vi "Adjust_Library_URL.vi"(8 "error in (no error)":errorcluster, 9 "libray ref":refnum<vi>, 10 "source path":path, 11 "Build in":refnum<class "AB_EXE.lvclass">) -> (0 "error out":errorcluster, 3 "Build out":refnum<class "AB_EXE.lvclass">)   [LabVIEW 2020, in "AB_EXE.lvclass"]
uses:
  <vilib>/AppBuilder/AB_Classes/EXE/AB_EXE.lvclass
  e:/builds/penguin/labview/branches/2020/dev/dist/vi.lib/AppBuilder/AB_Classes/Build/AB_Build.lvclass
  <vilib>/AppBuilder/AB_Classes/EXE/AB_EXE.lvclass/AB_EXE.ctl
  <vilib>/AppBuilder/AB_Classes/Build/AB_Build.lvclass
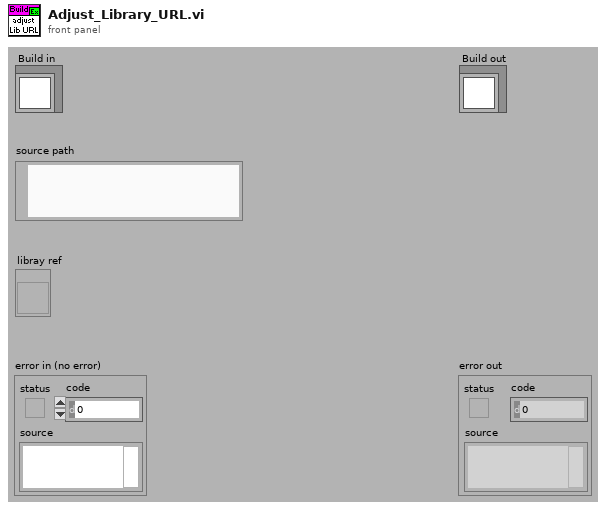
[diagram p1: front panel]
types:
  T1 = typedef "AB_EXE_SharedVar_LibInfo.ctl" = cluster{"LibraryPath":path, "LibraryItemID":string, "target":string, "deploy":bool}
  T2 = typedef "AB_Build.ctl" = cluster{"buildSpecName":string, "buildSpecDescription":string, "destinations":refnum<class "AB_Destination.lvclass">[], "exclusionOption":T3, "defaultLanguage":string, "supportedLanguages":string[], "excludedDirectories":path[], "buildContext":refnum<vi>, "buildObject":T4, "preview":bool, "programatic":bool, "progressBarEvents":T5, "userLog_Path":path, "preActionID":string, "preAction_Path":path, "postActionID":string, "postAction_Path":path, "eng_checkForBrokenVIs?":bool, "eng_verboseLinkerErrors?":bool, "localDest_Path":path, "targetDest_Path":path, "removeVIObject":u16, "cache":refnum<class "PreviewCache.lvclass">, "use cache":bool, "previewCache_ID":string, "buildCache_ID":string, "eng_TempLocalDest_Path":path, "eng_collectDependencies?":bool, "versionInfo":cluster{"buildVersion":cluster{"major":u16, "minor":u16, "patch":u16, "build":u16}, "autoIncrement":bool}, "eng_enableVIChecksums":bool}
  T3 = typedef "AB_Exclusion_Option.ctl" = cluster{"typedefs":bool, "polymorphicVIs":bool, "unusedLibraryItems":bool, "modifyLibraryFile":bool, "edit-timeDependencies":bool, "inlineVIs":bool, "dependent PPLs":bool, "dependent DLLs":bool}
  T4 = typedef "ItemRef.ctl" = u64
  T5 = typedef "provcom_ProgressBar_Events.ctl" = cluster{"newJob":refnum<user-event>, "newItem":refnum<user-event>, "errorMsg":T6, "cancel":refnum<user-event>}
  T6 = typedef "mxLvBuildError.ctl" = refnum<user-event>
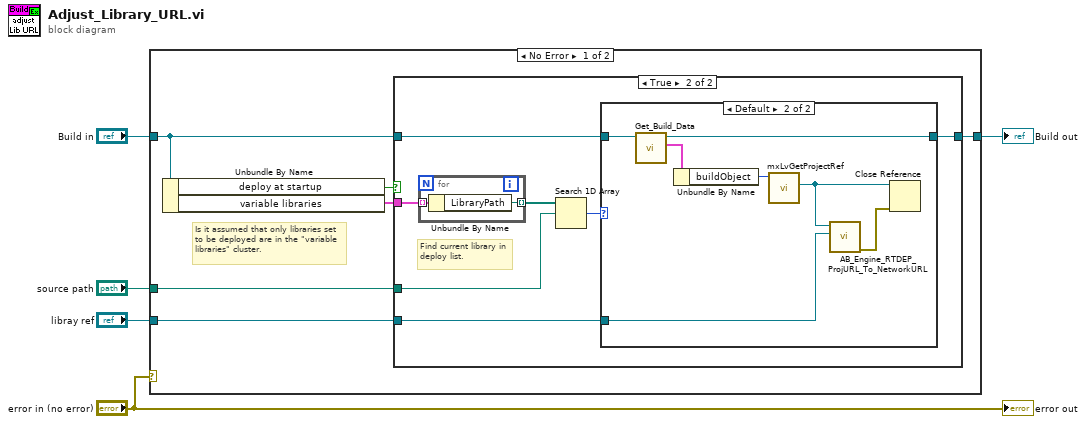
[diagram p0: block diagram]
diagram:
  n1 = case shown="No Error" "error in (no error)" {
    tunnel: "Build in" -> [w11 w30]
    tunnel: [w9 w30] -> w4
    tunnel: "source path" -> [w7 _]
    tunnel: "libray ref" -> [w6 _]
    frame No Error {
      # "Is it assumed that only libraries set to be deployed are in the \"variable libraries\" cluster."
      n2 = Unbundle By Name(w11) -> ("deploy at startup"=w10:bool, "variable libraries"=w8:T1[])
      n3 = case shown="True" w10 {
        tunnel: w11 -> [w12 w16]
        tunnel: [w12 w15] -> w9
        tunnel: w8 -> [_ w19]
        tunnel: w7 -> [_ w17]
        tunnel: w6 -> [_ w14]
        frame False {
        }
        frame True {
          # "Find current library in deploy list."
          n4 = for {
            tunnel: w19 -> [w29] mode=indexing
            tunnel: [w28] -> w18 mode=indexing
            n5 = Unbundle By Name(w29) -> ("LibraryPath"=w28:path)
          }
          n6 = Search 1D Array(1D array=w18, element=w17) -> (index of element=w13:i32)  [unwired: 1 out]
          n7 = case shown="Default" w13 {
            tunnel: w16 -> [w20 w27]
            tunnel: [w20 w26] -> w15
            tunnel: w14 -> [_ w21]
            frame -1 {
            }
            frame Default {
              n8 = call <vilib>:"Get_Build_Data.vi"("Class in"=w27) -> ("data"=w25:T2, "Class out"=w26:refnum<class "AB_EXE.lvclass">)  [unwired: 1 in, 8 out]
              n9 = Unbundle By Name(w25) -> ("buildObject"=w24:T4)
              n10 = call <resource>:"mxLvGetProjectRef.vi"("Item"=w24) -> ("Project Refnum"=w23:refnum<vi>)  [unwired: 1 in, 9 out]
              n11 = call <vilib>:"AB_Engine_RTDEP_ProjURL_To_NetworkURL.vi"("libray ref"=w21, "Project Refnum"=w23) -> ("error out"=w22:errorcluster)  [unwired: 1 in, 8 out]
              n12 = Close Reference(reference=w23, error in (no error)=w22) -> ()  [unwired: 1 out]
            }
          }
        }
      }
    }
    frame Error {
    }
  }
  "Build out" <- w4
  "error out" <- "error in (no error)"
